vi "BCU诊断标定.vi"(8 "CAN端口":u16(ring), 9 "设备索引号":u16(ring), 10 "CAN卡类型":u32(ring)=21, 11 "Myindex":dbl=1.0) -> (3 "成功":bool)   [LabVIEW 2013] (continued)
                                frame "SOH" {
                                n3888 = control-ref of="SOH(%)"() -> (w5508:refnum<vi>)
                                n3889 = property class="DigNum (严格)"(reference=w5508, "Value"=0.0 ("值")) -> ()  [unwired: 1 in, 2 out]
                                }
                                frame "一级故障阀值" {
                                n3890 = local write "一级故障"(T10 {"总电压过高"=0.0, "整组电压不均衡"=0.0, "SOC过高"=0.0, "单体电压过高"=0.0, "总电压过低"=0.0, "温度过高"=0.0, "温度过低"=0.0, "单组电压不均衡"=0.0, "整组温度不均衡"=0.0, "单组温度不均衡"=0.0, "单体电压过低"=0.0, "充电电流过高"=0.0, "放电电流过高"=0.0, "SOC过低"=0.0, "内阻过大"=0.0, "极柱温度过高"=0.0, "SOH过低"=0.0} ("一级故障")) -> ()
                                }
                                frame "二级故障阀值" {
                                n3891 = local write "一级故障 2"(T10 {"总电压过高"=0.0, "整组电压不均衡"=0.0, "SOC过高"=0.0, "单体电压过高"=0.0, "总电压过低"=0.0, "温度过高"=0.0, "温度过低"=0.0, "单组电压不均衡"=0.0, "整组温度不均衡"=0.0, "单组温度不均衡"=0.0, "单体电压过低"=0.0, "充电电流过高"=0.0, "放电电流过高"=0.0, "SOC过低"=0.0, "内阻过大"=0.0, "极柱温度过高"=0.0, "SOH过低"=0.0} ("一级故障")) -> ()
                                }
                                frame "三级故障阀值" {
                                n3892 = local write "一级故障 3"(T10 {"总电压过高"=0.0, "整组电压不均衡"=0.0, "SOC过高"=0.0, "单体电压过高"=0.0, "总电压过低"=0.0, "温度过高"=0.0, "温度过低"=0.0, "单组电压不均衡"=0.0, "整组温度不均衡"=0.0, "单组温度不均衡"=0.0, "单体电压过低"=0.0, "充电电流过高"=0.0, "放电电流过高"=0.0, "SOC过低"=0.0, "内阻过大"=0.0, "极柱温度过高"=0.0, "SOH过低"=0.0} ("一级故障")) -> ()
                                }
                                frame "加热控制参数" {
                                n3893 = local write "加热控制参数"(T11 {"风机开启温度"=0.0, "风机关闭温度"=0.0, "加热开启温度"=0.0, "加热关闭温度"=0.0, "风机开启温差"=0.0, "风机关闭温差"=0.0, "加热关闭温差"=0.0} ("加热控制参数")) -> ()
                                }
                                frame "充电控制参数" {
                                n3894 = local write "一级故障 5"(T12 {"最大允许单体电压"=0.0, "最大允许总电压"=0.0, "最小允许单体电压"=0.0, "最大允许充电电流"=0.0, "最小允许充电电流"=0.0, "最大允许充电温度"=0.0, "最小允许充电温度"=0.0, "电流步长"=0.0} ("一级故障 5")) -> ()
                                }
                                frame "电池信息1" {
                                w5514 = ""
                                w5515 = 0.0 ("电池串联")
                                n3895 = local read "电池信息"() -> (w5517:T13)
                                n3896 = Bundle By Name(cluster=w5517, "电池串联"=w5515, "电池并联"=w5515, "电池包额定容量"=w5515, "电池包额定能量(kWh)"=w5515, "电池包额定总电压"=w5515, "实际容量"=w5515, "电池厂家"=w5514, "电池类型"=w5514, "电池生产日期"=w5514) -> (w5516:T13)
                                n3897 = local write "电池信息"(w5516) -> ()
                                }
                                frame "电池包组号" {
                                n3898 = local read "电池信息"() -> (w5520:T13)
                                n3899 = Bundle By Name(cluster=w5520, "电池包组号"="") -> (w5519:T13)
                                n3900 = local write "电池信息"(w5519) -> ()
                                }
                                frame "充放电安时" {
                                w5521 = 0.0 ("累计充电总安时")
                                n3901 = local read "电池信息"() -> (w5523:T13)
                                n3902 = Bundle By Name(cluster=w5523, "累计充电总安时"=w5521, "累计放电总安时"=w5521) -> (w5522:T13)
                                n3903 = local write "电池信息"(w5522) -> ()
                                }
                                frame "电池充放电次数" {
                                w5524 = 0.0 ("累计充电总安时")
                                n3904 = local read "电池信息"() -> (w5526:T13)
                                n3905 = Bundle By Name(cluster=w5526, "电池充满次数"=w5524, "电池放空次数"=w5524, "电池充电次数"=w5524) -> (w5525:T13)
                                n3906 = local write "电池信息"(w5525) -> ()
                                }
                                }
                              }
                              frame "从板" {
                                n3907 = case shown="\"温度起始值\"" w5527 {
                                frame "假", Default {
                                }
                                frame "电压起始值" {
                                n3908 = for {
                                N: 1 -> [_]
                                tunnel: [""] -> w5532 mode=indexing
                                }
                                n3909 = control-ref of="项目信息 2"() -> (w5528:refnum<vi>)
                                n3910 = call "表格数据输入-8.6.vi"("行数"=u32 0, "列数"=u32 1, "字符串数组"=w5532, "表格引用"=w5528) -> ()  [unwired: 8 in]
                                }
                                frame "通道电压个数" {
                                n3911 = for {
                                N: 5 -> [_]
                                tunnel: [""] -> w5538 mode=indexing
                                }
                                n3912 = control-ref of="项目信息 2"() -> (w5534:refnum<vi>)
                                n3913 = call "表格数据输入-8.6.vi"("行数"=u32 22, "列数"=u32 1, "字符串数组"=w5538, "表格引用"=w5534) -> ()  [unwired: 8 in]
                                }
                                frame "保险位置" {
                                n3914 = for {
                                N: 10 -> [_]
                                tunnel: [""] -> w5544 mode=indexing
                                }
                                n3915 = control-ref of="项目信息 2"() -> (w5540:refnum<vi>)
                                n3916 = call "表格数据输入-8.6.vi"("行数"=u32 2, "列数"=u32 1, "字符串数组"=w5544, "表格引用"=w5540) -> ()  [unwired: 8 in]
                                }
                                frame "温度起始值" {
                                n3917 = for {
                                N: 1 -> [_]
                                tunnel: [""] -> w5550 mode=indexing
                                }
                                n3918 = control-ref of="项目信息 2"() -> (w5546:refnum<vi>)
                                n3919 = call "表格数据输入-8.6.vi"("行数"=u32 1, "列数"=u32 1, "字符串数组"=w5550, "表格引用"=w5546) -> ()  [unwired: 8 in]
                                }
                                frame "加热控制参数" {
                                n3920 = local write "加热控制参数"(T11 {"风机开启温度"=0.0, "风机关闭温度"=0.0, "加热开启温度"=0.0, "加热关闭温度"=0.0, "风机开启温差"=0.0, "风机关闭温差"=0.0, "加热关闭温差"=0.0} ("加热控制参数")) -> ()
                                }
                                frame "一级故障阀值" {
                                n3921 = local write "一级故障 6"(T15 {"电压过高"=0.0, "电压过低"=0.0, "温度过高"=0.0, "温度过低"=0.0, "电压不均衡(V)"=0.0, "温度不均衡"=0.0, "SOC过低"=0.0} ("一级故障 6")) -> ()
                                }
                                frame "二级故障阀值" {
                                n3922 = local write "一级故障 7"(T15 {"电压过高"=0.0, "电压过低"=0.0, "温度过高"=0.0, "温度过低"=0.0, "电压不均衡(V)"=0.0, "温度不均衡"=0.0, "SOC过低"=0.0} ("一级故障 7")) -> ()
                                }
                                frame "三级故障阀值" {
                                n3923 = local write "一级故障 8"(T15 {"电压过高"=0.0, "电压过低"=0.0, "温度过高"=0.0, "温度过低"=0.0, "电压不均衡(V)"=0.0, "温度不均衡"=0.0, "SOC过低"=0.0} ("一级故障 7")) -> ()
                                }
                                frame "均衡参数" {
                                n3924 = local write "均衡参数"(T17 {"充电结束电压(90%)"=0.0, "充电结束电压(91%)"=0.0, "充电结束电压(92%)"=0.0, "充电结束电压(93%)"=0.0, "充电结束电压(94%)"=0.0, "均衡计算-电压高阀值1级"=0.0, "均衡计算-电压高阀值2级"=0.0, "均衡计算-电压低阀值1级"=0.0, "均衡计算-电压低阀值2级"=0.0, "均衡计算-最低电压阀值"=0.0, "均衡停止-最低电压阀值"=0.0, "均衡计算-电压极差阀值"=0.0, "充电结束电压(95%)"=0.0, "充电结束电压(96%)"=0.0, "充电结束电压(97%)"=0.0, "充电结束电压(98%)"=0.0, "充电结束电压(99%)"=0.0, "充电结束电压(100%)"=0.0} ("均衡参数")) -> ()
                                }
                                frame "均衡阀值" {
                                w5557 = sgl 0.0 ("均衡计算-电压高阀值1级")
                                n3925 = local read "均衡参数"() -> (w5558:T17)
                                n3926 = Bundle By Name(cluster=w5558, "均衡计算-电压高阀值1级"=w5557, "均衡计算-电压高阀值2级"=w5557, "均衡计算-电压低阀值1级"=w5557, "均衡计算-电压低阀值2级"=w5557, "均衡计算-最低电压阀值"=w5557, "均衡停止-最低电压阀值"=w5557, "均衡计算-电压极差阀值"=w5557) -> (w5559:T17)
                                n3927 = local write "均衡参数"(w5559) -> ()
                                }
                                frame "充电结束电压" {
                                w5560 = sgl 0.0 ("均衡计算-电压高阀值1级")
                                n3928 = local read "均衡参数"() -> (w5561:T17)
                                n3929 = Bundle By Name(cluster=w5561, "充电结束电压(90%)"=w5560, "充电结束电压(91%)"=w5560, "充电结束电压(92%)"=w5560, "充电结束电压(93%)"=w5560, "充电结束电压(94%)"=w5560, "充电结束电压(95%)"=w5560, "充电结束电压(96%)"=w5560, "充电结束电压(97%)"=w5560, "充电结束电压(98%)"=w5560, "充电结束电压(99%)"=w5560, "充电结束电压(100%)"=w5560) -> (w5562:T17)
                                n3930 = local write "均衡参数"(w5562) -> ()
                                }
                                }
                              }
                            }
                          }
                          frame #1 {
                            w5563 = FALSE ("流控帧")
                            w5564 = TRUE ("流控帧 2")
                            n3931 = global write "EV05全局变量1.vi" "写入超时"(w5563) -> ()
                            n3932 = global write "EV05全局变量1.vi" "流控帧"(w5563) -> ()
                            n3933 = local write "写?"(w5563) -> ()
                            n3934 = local write "消除"(w5564) -> ()
                            n3935 = local write "控制1"(w5564) -> ()
                            n3936 = global write "EV05全局变量1.vi" "流控帧 2"(w5564) -> ()
                          }
                          frame #2 {
                            n3937 = Wait Until Next ms Multiple(millisecond multiple=u32 300 ("毫秒倍数")) -> ()  [unwired: 1 out]
                          }
                          frame #3 {
                            n3938 = local read "设备索引号"() -> (w5567:u16)
                            n3939 = local read "CAN卡类型"() -> (w5568:u32)
                            n3940 = local read "CAN端口"() -> (w5566:u16)
                            n3941 = local write "命令序号"(w5571) -> ()
                            n3942 = stacked-sequence {
                              tunnel: w5572 -> [_ w5579]
                              tunnel: w5571 -> [_ w5578]
                              tunnel: w5570 -> [_ w5577]
                              tunnel: w5569 -> [_ w5576]
                              tunnel: w5568 -> [_ w5575]
                              tunnel: w5567 -> [_ w5574]
                              tunnel: w5566 -> [_ w5573]
                              frame #0 {
                              }
                              frame #1 {
                                n3943 = call "多帧发送机制(EV05).vi"("can卡类型"=w5575, "设备索引号"=w5574, "CAN端口"=w5573, "命令"=w5579, "板号"=w5577, "命令序号"=w5578, "输入数据"=w5576) -> ()  [unwired: 2 in, 11 out]
                              }
                            }
                          }
                          frame #4 {
                            n3944 = while {
                              tunnel: [w5584] -> w5581
                              tunnel: [w5583] -> w5580
                              i -> [w5587]
                              stop <- w5584 stop-if-true
                              n3945 = local read "强制终止读写标记"() -> (w5582:bool)
                              n3946 = global read "EV05全局变量1.vi" "写入超时"() -> (w5583:bool)
                              n3947 = Greater Or Equal?(x=w5587, y=20) -> (x >= y?=w5585:bool)
                              n3948 = Compound Arithmetic op=OR(w5582, w5583, w5585) -> (w5584:bool)
                              n3949 = Wait Until Next ms Multiple(millisecond multiple=u32 100 ("毫秒倍数")) -> ()  [unwired: 1 out]
                            }
                          }
                          frame #5 {
                            n3950 = case shown="假" w5596 {
                              tunnel: w5595 -> [w5607 _]
                              tunnel: [w5602 w5619] -> w5594
                              tunnel: w5593 -> [w5601 _]
                              tunnel: w5592 -> [w5600 w5619]
                              tunnel: [w5599 w5618] -> w5589
                              tunnel: w5591 -> [w5598 _]
                              tunnel: w5590 -> [w5597 w5618]
                              frame False {
                                n3951 = local read "重试次数"() -> (w5606:u8)
                                n3952 = Increment(x=w5606) -> (x+1=w5605:u8)
                                n3953 = local write "重试次数"(w5605) -> ()
                                n3954 = Greater Or Equal?(x=w5605, y=u8 4) -> (x >= y?=w5604:bool)
                                n3955 = case shown="真" w5604 {
                                tunnel: w5607 -> [_ w5612]
                                tunnel: [w5609 w5611] -> w5602
                                tunnel: w5601 -> [w5609 _]
                                tunnel: w5600 -> [_ w5611]
                                tunnel: [w5608 w5610] -> w5599
                                tunnel: w5598 -> [w5608 _]
                                tunnel: w5597 -> [_ w5610]
                                frame False {
                                }
                                frame True {
                                n3956 = control-ref of="结果"() -> (w5614:refnum<vi>)
                                n3957 = Concatenate Strings(w5612, "     读取失败" ("字符串")) -> (w5616:string)
                                n3958 = Build Array(w5616) -> (w5613:string[])
                                n3959 = call "表格编辑.vi"("新元素/子数组"=w5613, "活动单元格:单元格背景色"=u32 16740749, "MCListbox引用句柄"=w5614) -> ()  [unwired: 9 out]
                                }
                                }
                              }
                              frame True {
                              }
                            }
                          }
                          frame #6 {
                            n3960 = And(x=w5621, y=w5623) -> (x .and. y?=w5622:bool)
                            n3961 = case shown="真" w5622 {
                              frame False {
                              }
                              frame True {
                                n3962 = local write "强制终止读写标记"(FALSE ("强制停止")) -> ()
                                n3963 = control-ref of="结果"() -> (w5626:refnum<vi>)
                                n3964 = Concatenate Strings("读取完成" ("字符串")) -> (w5628:string)
                                n3965 = Build Array(w5628) -> (w5625:string[])
                                n3966 = call "表格编辑.vi"("新元素/子数组"=w5625, "活动单元格:单元格背景色"=u32 21937, "MCListbox引用句柄"=w5626) -> ()  [unwired: 9 out]
                              }
                            }
                            n3967 = Wait (ms)(milliseconds to wait=u32 50 ("等待时间（毫秒）")) -> ()  [unwired: 1 out]
                          }
                        }
                      }
                    }
                  }
                  n3968 = local read "强制终止读写标记"() -> (w5394:bool)
                  n3969 = Or(x=w5394, y=w5393) -> (x .or. y?=w5391:bool)
                }
              }
            }
            frame #2 {
              n3970 = case shown="假" w5713 {
                tunnel: w5714 -> [w5715 _]
                frame False {
                  n3971 = case shown="\"主板\", 默认" w5715 {
                    frame "主板", Default {
                      n3972 = global read "读配置文件全局.vi" "电池额定实际容量判定"() -> (w5729:bool)
                      n3973 = global read "读配置文件全局.vi" "电池充放电次数判定"() -> (w5718:bool)
                      n3974 = global read "读配置文件全局.vi" "加热控制参数判定"() -> (w5716:bool)
                      n3975 = global read "读配置文件全局.vi" "配置文件版本判定"() -> (w5728:bool)
                      n3976 = global read "读配置文件全局.vi" "充电控制参数判定"() -> (w5722:bool)
                      n3977 = global read "读配置文件全局.vi" "通道电压数判定"() -> (w5734:bool)
                      n3978 = global read "读配置文件全局.vi" "电压起始值判定"() -> (w5733:bool)
                      n3979 = global read "读配置文件全局.vi" "温度起始值判定"() -> (w5731:bool)
                      n3980 = global read "读配置文件全局.vi" "充放电安时判定"() -> (w5720:bool)
                      n3981 = global read "读配置文件全局.vi" "电池包组号判定"() -> (w5719:bool)
                      n3982 = global read "读配置文件全局.vi" "电池信息1判定"() -> (w5721:bool)
                      n3983 = global read "读配置文件全局.vi" "从板个数判定"() -> (w5737:bool)
                      n3984 = global read "读配置文件全局.vi" "产品编号判定"() -> (w5736:bool)
                      n3985 = global read "读配置文件全局.vi" "电压个数判定"() -> (w5735:bool)
                      n3986 = global read "读配置文件全局.vi" "温度个数判定"() -> (w5732:bool)
                      n3987 = global read "读配置文件全局.vi" "保险位置判定"() -> (w5730:bool)
                      n3988 = global read "读配置文件全局.vi" "一级故障判定"() -> (w5725:bool)
                      n3989 = global read "读配置文件全局.vi" "二级故障判定"() -> (w5724:bool)
                      n3990 = global read "读配置文件全局.vi" "三级故障判定"() -> (w5723:bool)
                      n3991 = global read "读配置文件全局.vi" "车牌号判定"() -> (w5727:bool)
                      n3992 = global read "读配置文件全局.vi" "SOH判定"() -> (w5726:bool)
                      n3993 = Build Array(w5737, w5736, w5735, w5734, w5733, w5732, w5731, w5730, w5729, w5728, w5727, w5726, w5725, w5724, w5723, w5722, w5721, w5720, w5719, w5718, w5716) -> (w5717:bool[])
                      n3994 = And Array Elements(Boolean array=w5717) -> (logical AND=w5738:bool)
                      n3995 = disable-structure shown="禁用" {
                        frame Disabled {
                          n3996 = global read "读配置文件全局.vi" "SOC判定"() -> ()  [unwired: 1 out]
                        }
                        frame Enabled {
                        }
                      }
                      n3997 = case shown="假" w5738 {
                        tunnel: w5717 -> [_ w5743]
                        frame True {
                          n3998 = control-ref of="结果"() -> (w5741:refnum<vi>)
                          n3999 = Build Array("全部判定成功!!!!!!!!") -> (w5742:string[])
                          n4000 = call "表格编辑.vi"("新元素/子数组"=w5742, "活动单元格:单元格背景色"=u32 6618880, "MCListbox引用句柄"=w5741) -> ()  [unwired: 9 out]
                        }
                        frame False {
                          n4001 = stacked-sequence {
                            tunnel: w5743 -> [_ w5748]
                            frame #0 {
                              n4002 = control-ref of="结果"() -> (w5746:refnum<vi>)
                              n4003 = Build Array("全部判定失败!!!!!") -> (w5747:string[])
                              n4004 = call "表格编辑.vi"("新元素/子数组"=w5747, "活动单元格:单元格背景色"=u32 16711680, "MCListbox引用句柄"=w5746) -> ()  [unwired: 9 out]
                            }
                            frame #1 {
                              n4005 = for {
                                tunnel: w5748 -> [w5750] mode=indexing
                                i -> [w5749]
                                n4006 = case shown="20" w5749 {
                                tunnel: w5750 -> [w5751 w5756 w5761 w5766 w5771 w5776 w5781 w5786 w5791 w5796 w5801 w5806 w5811 w5816 w5821 w5826 w5831 w5836 w5841 w5846 w5851 _]
                                frame 0 {
                                n4007 = case shown="假" w5751 {
                                frame False {
                                n4008 = control-ref of="结果"() -> (w5754:refnum<vi>)
                                n4009 = Build Array("从板个数判定失败!") -> (w5755:string[])
                                n4010 = call "表格编辑.vi"("新元素/子数组"=w5755, "活动单元格:单元格背景色"=u32 16711680, "MCListbox引用句柄"=w5754) -> ()  [unwired: 9 out]
                                }
                                frame True {
                                }
                                }
                                }
                                frame 1 {
                                n4011 = case shown="假" w5756 {
                                frame False {
                                n4012 = control-ref of="结果"() -> (w5759:refnum<vi>)
                                n4013 = Build Array("产品编号判定失败!") -> (w5760:string[])
                                n4014 = call "表格编辑.vi"("新元素/子数组"=w5760, "活动单元格:单元格背景色"=u32 16711680, "MCListbox引用句柄"=w5759) -> ()  [unwired: 9 out]
                                }
                                frame True {
                                }
                                }
                                }
                                frame 2 {
                                n4015 = case shown="假" w5761 {
                                frame False {
                                n4016 = control-ref of="结果"() -> (w5764:refnum<vi>)
                                n4017 = Build Array("电压个数判定失败!") -> (w5765:string[])
                                n4018 = call "表格编辑.vi"("新元素/子数组"=w5765, "活动单元格:单元格背景色"=u32 16711680, "MCListbox引用句柄"=w5764) -> ()  [unwired: 9 out]
                                }
                                frame True {
                                }
                                }
                                }
                                frame 3 {
                                n4019 = case shown="假" w5766 {
                                frame False {
                                n4020 = control-ref of="结果"() -> (w5769:refnum<vi>)
                                n4021 = Build Array("通道电压数判定失败!") -> (w5770:string[])
                                n4022 = call "表格编辑.vi"("新元素/子数组"=w5770, "活动单元格:单元格背景色"=u32 16711680, "MCListbox引用句柄"=w5769) -> ()  [unwired: 9 out]
                                }
                                frame True {
                                }
                                }
                                }
                                frame 4 {
                                n4023 = case shown="假" w5771 {
                                frame False {
                                n4024 = control-ref of="结果"() -> (w5774:refnum<vi>)
                                n4025 = Build Array("电压起始值判定失败!") -> (w5775:string[])
                                n4026 = call "表格编辑.vi"("新元素/子数组"=w5775, "活动单元格:单元格背景色"=u32 16711680, "MCListbox引用句柄"=w5774) -> ()  [unwired: 9 out]
                                }
                                frame True {
                                }
                                }
                                }
                                frame 5 {
                                n4027 = case shown="假" w5776 {
                                frame False {
                                n4028 = control-ref of="结果"() -> (w5779:refnum<vi>)
                                n4029 = Build Array("温度个数判定失败!") -> (w5780:string[])
                                n4030 = call "表格编辑.vi"("新元素/子数组"=w5780, "活动单元格:单元格背景色"=u32 16711680, "MCListbox引用句柄"=w5779) -> ()  [unwired: 9 out]
                                }
                                frame True {
                                }
                                }
                                }
                                frame 6 {
                                n4031 = case shown="假" w5781 {
                                frame False {
                                n4032 = control-ref of="结果"() -> (w5784:refnum<vi>)
                                n4033 = Build Array("温度起始值判定失败!") -> (w5785:string[])
                                n4034 = call "表格编辑.vi"("新元素/子数组"=w5785, "活动单元格:单元格背景色"=u32 16711680, "MCListbox引用句柄"=w5784) -> ()  [unwired: 9 out]
                                }
                                frame True {
                                }
                                }
                                }
                                frame 7 {
                                n4035 = case shown="假" w5786 {
                                frame False {
                                n4036 = control-ref of="结果"() -> (w5789:refnum<vi>)
                                n4037 = Build Array("保险位置判定失败!") -> (w5790:string[])
                                n4038 = call "表格编辑.vi"("新元素/子数组"=w5790, "活动单元格:单元格背景色"=u32 16711680, "MCListbox引用句柄"=w5789) -> ()  [unwired: 9 out]
                                }
                                frame True {
                                }
                                }
                                }
                                frame 8 {
                                n4039 = case shown="假" w5791 {
                                frame False {
                                n4040 = control-ref of="结果"() -> (w5794:refnum<vi>)
                                n4041 = Build Array("电池额定实际容量判定失败!") -> (w5795:string[])
                                n4042 = call "表格编辑.vi"("新元素/子数组"=w5795, "活动单元格:单元格背景色"=u32 16711680, "MCListbox引用句柄"=w5794) -> ()  [unwired: 9 out]
                                }
                                frame True {
                                }
                                }
                                }
                                frame 9 {
                                n4043 = case shown="假" w5796 {
                                frame False {
                                n4044 = control-ref of="结果"() -> (w5799:refnum<vi>)
                                n4045 = Build Array("配置文件版本判定失败!") -> (w5800:string[])
                                n4046 = call "表格编辑.vi"("新元素/子数组"=w5800, "活动单元格:单元格背景色"=u32 16711680, "MCListbox引用句柄"=w5799) -> ()  [unwired: 9 out]
                                }
                                frame True {
                                }
                                }
                                }
                                frame 10 {
                                n4047 = case shown="假" w5801 {
                                frame False {
                                n4048 = control-ref of="结果"() -> (w5804:refnum<vi>)
                                n4049 = Build Array("车牌号判定失败!") -> (w5805:string[])
                                n4050 = call "表格编辑.vi"("新元素/子数组"=w5805, "活动单元格:单元格背景色"=u32 16711680, "MCListbox引用句柄"=w5804) -> ()  [unwired: 9 out]
                                }
                                frame True {
                                }
                                }
                                }
                                frame 11 {
                                n4051 = case shown="假" w5806 {
                                frame False {
                                n4052 = control-ref of="结果"() -> (w5809:refnum<vi>)
                                n4053 = Build Array("SOH判定失败!") -> (w5810:string[])
                                n4054 = call "表格编辑.vi"("新元素/子数组"=w5810, "活动单元格:单元格背景色"=u32 16711680, "MCListbox引用句柄"=w5809) -> ()  [unwired: 9 out]
                                }
                                frame True {
                                }
                                }
                                }
                                frame 12 {
                                n4055 = case shown="假" w5811 {
                                frame False {
                                n4056 = control-ref of="结果"() -> (w5814:refnum<vi>)
                                n4057 = Build Array("一级故障阀值判定失败!") -> (w5815:string[])
                                n4058 = call "表格编辑.vi"("新元素/子数组"=w5815, "活动单元格:单元格背景色"=u32 16711680, "MCListbox引用句柄"=w5814) -> ()  [unwired: 9 out]
                                }
                                frame True {
                                }
                                }
                                }
                                frame 13 {
                                n4059 = case shown="假" w5816 {
                                frame False {
                                n4060 = control-ref of="结果"() -> (w5819:refnum<vi>)
                                n4061 = Build Array("二级故障阀值判定失败!") -> (w5820:string[])
                                n4062 = call "表格编辑.vi"("新元素/子数组"=w5820, "活动单元格:单元格背景色"=u32 16711680, "MCListbox引用句柄"=w5819) -> ()  [unwired: 9 out]
                                }
                                frame True {
                                }
                                }
                                }
                                frame 14 {
                                n4063 = case shown="假" w5821 {
                                frame False {
                                n4064 = control-ref of="结果"() -> (w5824:refnum<vi>)
                                n4065 = Build Array("三级故障阀值判定失败!") -> (w5825:string[])
                                n4066 = call "表格编辑.vi"("新元素/子数组"=w5825, "活动单元格:单元格背景色"=u32 16711680, "MCListbox引用句柄"=w5824) -> ()  [unwired: 9 out]
                                }
                                frame True {
                                }
                                }
                                }
                                frame 15 {
                                n4067 = case shown="假" w5826 {
                                frame False {
                                n4068 = control-ref of="结果"() -> (w5829:refnum<vi>)
                                n4069 = Build Array("充电控制参数判定失败!") -> (w5830:string[])
                                n4070 = call "表格编辑.vi"("新元素/子数组"=w5830, "活动单元格:单元格背景色"=u32 16711680, "MCListbox引用句柄"=w5829) -> ()  [unwired: 9 out]
                                }
                                frame True {
                                }
                                }
                                }
                                frame 16 {
                                n4071 = case shown="假" w5831 {
                                frame False {
                                n4072 = control-ref of="结果"() -> (w5834:refnum<vi>)
                                n4073 = Build Array("电池信息1判定失败!") -> (w5835:string[])
                                n4074 = call "表格编辑.vi"("新元素/子数组"=w5835, "活动单元格:单元格背景色"=u32 16711680, "MCListbox引用句柄"=w5834) -> ()  [unwired: 9 out]
                                }
                                frame True {
                                }
                                }
                                }
                                frame 17 {
                                n4075 = case shown="假" w5836 {
                                frame False {
                                n4076 = control-ref of="结果"() -> (w5839:refnum<vi>)
                                n4077 = Build Array("充放电安时判定失败!") -> (w5840:string[])
                                n4078 = call "表格编辑.vi"("新元素/子数组"=w5840, "活动单元格:单元格背景色"=u32 16711680, "MCListbox引用句柄"=w5839) -> ()  [unwired: 9 out]
                                }
                                frame True {
                                }
                                }
                                }
                                frame 18 {
                                n4079 = case shown="假" w5841 {
                                frame False {
                                n4080 = control-ref of="结果"() -> (w5844:refnum<vi>)
                                n4081 = Build Array("电池包组号判定失败!") -> (w5845:string[])
                                n4082 = call "表格编辑.vi"("新元素/子数组"=w5845, "活动单元格:单元格背景色"=u32 16711680, "MCListbox引用句柄"=w5844) -> ()  [unwired: 9 out]
                                }
                                frame True {
                                }
                                }
                                }
                                frame 19 {
                                n4083 = case shown="假" w5846 {
                                frame False {
                                n4084 = control-ref of="结果"() -> (w5849:refnum<vi>)
                                n4085 = Build Array("电池充放电次数判定失败!") -> (w5850:string[])
                                n4086 = call "表格编辑.vi"("新元素/子数组"=w5850, "活动单元格:单元格背景色"=u32 16711680, "MCListbox引用句柄"=w5849) -> ()  [unwired: 9 out]
                                }
                                frame True {
                                }
                                }
                                }
                                frame 20 {
                                n4087 = case shown="假" w5851 {
                                frame False {
                                n4088 = control-ref of="结果"() -> (w5854:refnum<vi>)
                                n4089 = Build Array("加热控制参数判定失败!") -> (w5855:string[])
                                n4090 = call "表格编辑.vi"("新元素/子数组"=w5855, "活动单元格:单元格背景色"=u32 16711680, "MCListbox引用句柄"=w5854) -> ()  [unwired: 9 out]
                                }
                                frame True {
                                }
                                }
                                }
                                frame 99, Default {
                                }
                                }
                              }
                            }
                          }
                        }
                      }
                    }
                    frame "从板" {
                      n4091 = global read "读配置文件全局2.vi" "电压起始值判定"() -> (w5864:bool)
                      n4092 = global read "读配置文件全局2.vi" "温度起始值判定"() -> (w5861:bool)
                      n4093 = global read "读配置文件全局2.vi" "加热控制参数判定"() -> (w5856:bool)
                      n4094 = global read "读配置文件全局2.vi" "通道电压判定"() -> (w5863:bool)
                      n4095 = global read "读配置文件全局2.vi" "保险位置判定"() -> (w5862:bool)
                      n4096 = global read "读配置文件全局2.vi" "一级故障判定"() -> (w5859:bool)
                      n4097 = global read "读配置文件全局2.vi" "二级故障判定"() -> (w5858:bool)
                      n4098 = global read "读配置文件全局2.vi" "三级故障判定"() -> (w5857:bool)
                      n4099 = global read "读配置文件全局2.vi" "从板号判定"() -> (w5865:bool)
                      n4100 = Build Array(w5865, w5864, w5863, w5862, w5861, w5859, w5858, w5857, w5856) -> (w5860:bool[])
                      n4101 = And Array Elements(Boolean array=w5860) -> (logical AND=w5866:bool)
                      n4102 = case shown="假" w5866 {
                        tunnel: w5860 -> [_ w5871]
                        frame True {
                          n4103 = control-ref of="结果"() -> (w5869:refnum<vi>)
                          n4104 = Build Array("读取判定成功!!!!!!!!") -> (w5870:string[])
                          n4105 = call "表格编辑.vi"("新元素/子数组"=w5870, "活动单元格:单元格背景色"=u32 6618880, "MCListbox引用句柄"=w5869) -> ()  [unwired: 9 out]
                        }
                        frame False {
                          n4106 = stacked-sequence {
                            tunnel: w5871 -> [_ w5876]
                            frame #0 {
                              n4107 = control-ref of="结果"() -> (w5874:refnum<vi>)
                              n4108 = Build Array("读取判定失败!!!!!") -> (w5875:string[])
                              n4109 = call "表格编辑.vi"("新元素/子数组"=w5875, "活动单元格:单元格背景色"=u32 16711680, "MCListbox引用句柄"=w5874) -> ()  [unwired: 9 out]
                            }
                            frame #1 {
                              n4110 = for {
                                tunnel: w5876 -> [w5877] mode=indexing
                                i -> [w5878]
                                n4111 = case shown="0" w5878 {
                                tunnel: w5877 -> [w5879 w5884 w5889 w5894 w5899 w5904 w5909 w5914 w5919 _]
                                frame 0 {
                                n4112 = case shown="假" w5879 {
                                frame False {
                                n4113 = control-ref of="结果"() -> (w5882:refnum<vi>)
                                n4114 = Build Array("从板号判定失败!") -> (w5883:string[])
                                n4115 = call "表格编辑.vi"("新元素/子数组"=w5883, "活动单元格:单元格背景色"=u32 16711680, "MCListbox引用句柄"=w5882) -> ()  [unwired: 9 out]
                                }
                                frame True {
                                }
                                }
                                }
                                frame 1 {
                                n4116 = case shown="假" w5884 {
                                frame False {
                                n4117 = control-ref of="结果"() -> (w5887:refnum<vi>)
                                n4118 = Build Array("电压起始值判定失败!") -> (w5888:string[])
                                n4119 = call "表格编辑.vi"("新元素/子数组"=w5888, "活动单元格:单元格背景色"=u32 16711680, "MCListbox引用句柄"=w5887) -> ()  [unwired: 9 out]
                                }
                                frame True {
                                }
                                }
                                }
                                frame 2 {
                                n4120 = case shown="假" w5889 {
                                frame False {
                                n4121 = control-ref of="结果"() -> (w5892:refnum<vi>)
                                n4122 = Build Array("通道电压节数判定失败!") -> (w5893:string[])
                                n4123 = call "表格编辑.vi"("新元素/子数组"=w5893, "活动单元格:单元格背景色"=u32 16711680, "MCListbox引用句柄"=w5892) -> ()  [unwired: 9 out]
                                }
                                frame True {
                                }
                                }
                                }
                                frame 3 {
                                n4124 = case shown="假" w5894 {
                                frame False {
                                n4125 = control-ref of="结果"() -> (w5897:refnum<vi>)
                                n4126 = Build Array("保险位置判定失败!") -> (w5898:string[])
                                n4127 = call "表格编辑.vi"("新元素/子数组"=w5898, "活动单元格:单元格背景色"=u32 16711680, "MCListbox引用句柄"=w5897) -> ()  [unwired: 9 out]
                                }
                                frame True {
                                }
                                }
                                }
                                frame 4 {
                                n4128 = case shown="假" w5899 {
                                frame False {
                                n4129 = control-ref of="结果"() -> (w5902:refnum<vi>)
                                n4130 = Build Array("温度起始值判定失败!") -> (w5903:string[])
                                n4131 = call "表格编辑.vi"("新元素/子数组"=w5903, "活动单元格:单元格背景色"=u32 16711680, "MCListbox引用句柄"=w5902) -> ()  [unwired: 9 out]
                                }
                                frame True {
                                }
                                }
                                }
                                frame 5 {
                                n4132 = case shown="假" w5904 {
                                frame False {
                                n4133 = control-ref of="结果"() -> (w5907:refnum<vi>)
                                n4134 = Build Array("一级故障判定失败!") -> (w5908:string[])
                                n4135 = call "表格编辑.vi"("新元素/子数组"=w5908, "活动单元格:单元格背景色"=u32 16711680, "MCListbox引用句柄"=w5907) -> ()  [unwired: 9 out]
                                }
                                frame True {
                                }
                                }
                                }
                                frame 6 {
                                n4136 = case shown="假" w5909 {
                                frame False {
                                n4137 = control-ref of="结果"() -> (w5912:refnum<vi>)
                                n4138 = Build Array("二级故障判定失败!") -> (w5913:string[])
                                n4139 = call "表格编辑.vi"("新元素/子数组"=w5913, "活动单元格:单元格背景色"=u32 16711680, "MCListbox引用句柄"=w5912) -> ()  [unwired: 9 out]
                                }
                                frame True {
                                }
                                }
                                }
                                frame 7 {
                                n4140 = case shown="假" w5914 {
                                frame False {
                                n4141 = control-ref of="结果"() -> (w5917:refnum<vi>)
                                n4142 = Build Array("三级故障判定失败!") -> (w5918:string[])
                                n4143 = call "表格编辑.vi"("新元素/子数组"=w5918, "活动单元格:单元格背景色"=u32 16711680, "MCListbox引用句柄"=w5917) -> ()  [unwired: 9 out]
                                }
                                frame True {
                                }
                                }
                                }
                                frame 8 {
                                n4144 = case shown="假" w5919 {
                                frame False {
                                n4145 = control-ref of="结果"() -> (w5922:refnum<vi>)
                                n4146 = Build Array("加热控制参数判定失败!") -> (w5923:string[])
                                n4147 = call "表格编辑.vi"("新元素/子数组"=w5923, "活动单元格:单元格背景色"=u32 16711680, "MCListbox引用句柄"=w5922) -> ()  [unwired: 9 out]
                                }
                                frame True {
                                }
                                }
                                }
                                frame 99, Default {
                                }
                                }
                              }
                            }
                          }
                        }
                      }
                      n4148 = disable-structure shown="禁用" {
                        frame Disabled {
                          n4149 = global read "读配置文件全局.vi" "SOC判定"() -> ()  [unwired: 1 out]
                        }
                        frame Enabled {
                        }
                      }
                    }
                  }
                }
                frame True {
                }
              }
            }
          }
          n4150 = stacked-sequence {
            tunnel: w5156 -> [_]
            frame #0 {
              n4151 = local write "强制终止读写标记"(FALSE ("强制停止")) -> ()
            }
          }
          "重试次数" <- u8 0 ("重试次数")
        }
        frame "开启均衡" {
          n4152 = local read "从板板号"() -> (w5924:u8)
          n4153 = stacked-sequence {
            tunnel: 133 -> [_ w5950 _ _]
            tunnel: w5924 -> [_ _ _ _]
            frame #0 {
              w5934 = u8 0 items=["Normal", "Listen Only"] ("工作方式")
              w5933 = u8 1 items=["Dual Filter", "Single Filter"] ("滤波方式")
              n4154 = global write "EV05全局变量1.vi" "读取超时"(FALSE ("读取超时")) -> ()
              n4155 = global write "EV05全局变量1.vi" "流控帧 2"(TRUE ("流控帧 2")) -> ()
              n4156 = local write "写?"(TRUE ("写?")) -> ()
              n4157 = local read "设备索引号"() -> (w5929:u16)
              n4158 = local read "CAN卡类型"() -> (w5928:u32)
              n4159 = local read "CAN端口"() -> (w5930:u16)
              n4160 = local write "控制1"(TRUE ("控制1")) -> ()
              n4161 = local write "消除"(TRUE ("消除")) -> ()
              n4162 = global write "EV05全局变量1.vi" "流控帧"(FALSE ("流控帧")) -> ()
              n4163 = call "CAN_Init-8.6.vi"("CAN卡类型"=w5928, "设备索引号"=w5929, "CAN端口"=w5930, "操作类型"=enum16{"初始化CAN", "关闭CAN"}."初始化CAN", "滤波方式"=w5933, "Accept Code"=u32 606601216, "簇"=T23 {"打开CAN"=FALSE, "初始化CAN"=TRUE, "开始CAN"=TRUE, "重启"=FALSE, "关闭CAN"=FALSE}, "Mask Code"=u32 524287 ("Accept Code"), "工作方式"=w5934, "是否滤波"=TRUE, "滤波选择"=T22 {"fiter_mode"=1, "fiter_endid"=75825152, "fiter_startid"=75890687}) -> ()  [unwired: 3 in, 6 out]
              n4164 = Wait Until Next ms Multiple(millisecond multiple=u32 20 ("毫秒倍数")) -> ()  [unwired: 1 out]
            }
            frame #1 {
              n4165 = local write "命令"(w5950) -> ()
              n4166 = call "ID组合.vi"("SA(4)"=0 ("PDU(1)"), "PS(3)"=63 ("PDU(1)"), "PF(2)"=w5950, "PDU(1)"=4) -> ("ID"=w5949:i32)  [unwired: 7 out]
              n4167 = local read "均衡类型选择"() -> (w5946:enum16{"放电均衡", "充电均衡", "充放电均衡"})
              n4168 = local read "设备索引号"() -> (w5955:u16)
              n4169 = local read "CAN卡类型"() -> (w5956:u32)
              n4170 = local read "CAN端口"() -> (w5954:u16)
              n4171 = local write "命令序号"(2) -> ()
              n4172 = Add(x=w5946, y=1) -> (x+y=w5944:i32)
              n4173 = Build Array(2, 2, w5944) -> (w5957:i32[])
              n4174 = call "transmit-8.6.vi"("can卡类型"=w5956, "设备索引号"=w5955, "CAN端口"=w5954, "ID"=w5949, "SendType"=u8 0, "Data"=w5957) -> ()  [unwired: 3 in, 11 out]
            }
            frame #2 {
              n4175 = Wait Until Next ms Multiple(millisecond multiple=u32 1000 ("毫秒倍数")) -> ()  [unwired: 1 out]
            }
            frame #3 {
              w5965 = u8 0 items=["Normal", "Listen Only"] ("工作方式")
              w5966 = u8 1 items=["Dual Filter", "Single Filter"] ("滤波方式")
              n4176 = global write "EV05全局变量1.vi" "流控帧 2"(FALSE ("流控帧 2")) -> ()
              n4177 = local read "CAN卡类型"() -> (w5971:u32)
              n4178 = local read "设备索引号"() -> (w5970:u16)
              n4179 = local read "CAN端口"() -> (w5969:u16)
              n4180 = local write "控制1"(FALSE ("控制1")) -> ()
              n4181 = local write "消除"(FALSE ("消除")) -> ()
              n4182 = call <vilib>:"Unset Busy.vi"() -> ()  [unwired: 2 in, 10 out]
              n4183 = call "CAN_Init-8.6.vi"("CAN卡类型"=w5971, "设备索引号"=w5970, "CAN端口"=w5969, "操作类型"=enum16{"初始化CAN", "关闭CAN"}."初始化CAN", "滤波方式"=w5966, "Accept Code"=u32 3221225472, "簇"=T23 {"打开CAN"=FALSE, "初始化CAN"=TRUE, "开始CAN"=TRUE, "重启"=FALSE, "关闭CAN"=FALSE}, "Mask Code"=u32 1073741823 ("Accept Code"), "工作方式"=w5965, "是否滤波"=TRUE, "滤波选择"=T22 {"fiter_mode"=1, "fiter_endid"=402653184, "fiter_startid"=419430399}) -> ()  [unwired: 3 in, 6 out]
            }
          }
        }
        frame "关闭均衡" {
          n4184 = local read "从板板号"() -> (w5975:u8)
          n4185 = stacked-sequence {
            tunnel: 133 -> [_ w5999 _ _]
            tunnel: w5975 -> [_ _ _ _]
            frame #0 {
              w5985 = u8 0 items=["Normal", "Listen Only"] ("工作方式")
              w5984 = u8 1 items=["Dual Filter", "Single Filter"] ("滤波方式")
              n4186 = global write "EV05全局变量1.vi" "读取超时"(FALSE ("读取超时")) -> ()
              n4187 = global write "EV05全局变量1.vi" "流控帧 2"(TRUE ("流控帧 2")) -> ()
              n4188 = local write "写?"(TRUE ("写?")) -> ()
              n4189 = local read "设备索引号"() -> (w5980:u16)
              n4190 = local read "CAN卡类型"() -> (w5979:u32)
              n4191 = local read "CAN端口"() -> (w5981:u16)
              n4192 = local write "控制1"(TRUE ("控制1")) -> ()
              n4193 = global write "EV05全局变量1.vi" "流控帧"(FALSE ("流控帧")) -> ()
              n4194 = local write "消除"(TRUE ("消除")) -> ()
              n4195 = call "CAN_Init-8.6.vi"("CAN卡类型"=w5979, "设备索引号"=w5980, "CAN端口"=w5981, "操作类型"=enum16{"初始化CAN", "关闭CAN"}."初始化CAN", "滤波方式"=w5984, "Accept Code"=u32 606601216, "簇"=T23 {"打开CAN"=FALSE, "初始化CAN"=TRUE, "开始CAN"=TRUE, "重启"=FALSE, "关闭CAN"=FALSE}, "Mask Code"=u32 524287 ("Accept Code"), "工作方式"=w5985, "是否滤波"=TRUE, "滤波选择"=T22 {"fiter_mode"=1, "fiter_endid"=75825152, "fiter_startid"=75890687}) -> ()  [unwired: 3 in, 6 out]
              n4196 = Wait Until Next ms Multiple(millisecond multiple=u32 20 ("毫秒倍数")) -> ()  [unwired: 1 out]
            }
            frame #1 {
              n4197 = local write "命令"(w5999) -> ()
              n4198 = call "ID组合.vi"("SA(4)"=0 ("PDU(1)"), "PS(3)"=63 ("PDU(1)"), "PF(2)"=w5999, "PDU(1)"=4) -> ("ID"=w5998:i32)  [unwired: 7 out]
              n4199 = local read "均衡类型选择"() -> (w6009:enum16{"放电均衡", "充电均衡", "充放电均衡"})
              n4200 = local write "命令序号"(3) -> ()
              n4201 = local read "设备索引号"() -> (w6004:u16)
              n4202 = local read "CAN卡类型"() -> (w6005:u32)
              n4203 = local read "CAN端口"() -> (w6003:u16)
              n4204 = Add(x=w6009, y=1) -> (x+y=w6007:i32)
              n4205 = Build Array(2, 3, w6007) -> (w6006:i32[])
              n4206 = call "transmit-8.6.vi"("can卡类型"=w6005, "设备索引号"=w6004, "CAN端口"=w6003, "ID"=w5998, "SendType"=u8 0, "Data"=w6006) -> ()  [unwired: 3 in, 11 out]
            }
            frame #2 {
              n4207 = Wait Until Next ms Multiple(millisecond multiple=u32 1000 ("毫秒倍数")) -> ()  [unwired: 1 out]
            }
            frame #3 {
              w6016 = u8 0 items=["Normal", "Listen Only"] ("工作方式")
              w6017 = u8 1 items=["Dual Filter", "Single Filter"] ("滤波方式")
              n4208 = local read "设备索引号"() -> (w6021:u16)
              n4209 = local read "CAN卡类型"() -> (w6022:u32)
              n4210 = global write "EV05全局变量1.vi" "流控帧 2"(FALSE ("流控帧 2")) -> ()
              n4211 = local read "CAN端口"() -> (w6020:u16)
              n4212 = local write "控制1"(FALSE ("控制1")) -> ()
              n4213 = local write "消除"(FALSE ("消除")) -> ()
              n4214 = call "CAN_Init-8.6.vi"("CAN卡类型"=w6022, "设备索引号"=w6021, "CAN端口"=w6020, "操作类型"=enum16{"初始化CAN", "关闭CAN"}."初始化CAN", "滤波方式"=w6017, "Accept Code"=u32 3221225472, "簇"=T23 {"打开CAN"=FALSE, "初始化CAN"=TRUE, "开始CAN"=TRUE, "重启"=FALSE, "关闭CAN"=FALSE}, "Mask Code"=u32 1073741823 ("Accept Code"), "工作方式"=w6016, "是否滤波"=TRUE, "滤波选择"=T22 {"fiter_mode"=1, "fiter_endid"=402653184, "fiter_startid"=419430399}) -> ()  [unwired: 3 in, 6 out]
              n4215 = call <vilib>:"Unset Busy.vi"() -> ()  [unwired: 2 in, 10 out]
            }
          }
        }
        frame "强制均衡" {
          n4216 = local read "从板板号"() -> (w6026:u8)
          n4217 = stacked-sequence {
            tunnel: 133 -> [_ w6057 _ _]
            tunnel: w6026 -> [_ _ _ _]
            frame #0 {
              w6036 = u8 0 items=["Normal", "Listen Only"] ("工作方式")
              w6035 = u8 1 items=["Dual Filter", "Single Filter"] ("滤波方式")
              n4218 = global write "EV05全局变量1.vi" "读取超时"(FALSE ("读取超时")) -> ()
              n4219 = global write "EV05全局变量1.vi" "流控帧 2"(TRUE ("流控帧 2")) -> ()
              n4220 = local write "写?"(TRUE ("写?")) -> ()
              n4221 = local read "设备索引号"() -> (w6031:u16)
              n4222 = local read "CAN卡类型"() -> (w6030:u32)
              n4223 = local write "控制1"(TRUE ("控制1")) -> ()
              n4224 = local read "CAN端口"() -> (w6032:u16)
              n4225 = local write "消除"(TRUE ("消除")) -> ()
              n4226 = global write "EV05全局变量1.vi" "流控帧"(FALSE ("流控帧")) -> ()
              n4227 = call "CAN_Init-8.6.vi"("CAN卡类型"=w6030, "设备索引号"=w6031, "CAN端口"=w6032, "操作类型"=enum16{"初始化CAN", "关闭CAN"}."初始化CAN", "滤波方式"=w6035, "Accept Code"=u32 606601216, "簇"=T23 {"打开CAN"=FALSE, "初始化CAN"=TRUE, "开始CAN"=TRUE, "重启"=FALSE, "关闭CAN"=FALSE}, "Mask Code"=u32 524287 ("Accept Code"), "工作方式"=w6036, "是否滤波"=TRUE, "滤波选择"=T22 {"fiter_mode"=1, "fiter_endid"=75825152, "fiter_startid"=75890687}) -> ()  [unwired: 3 in, 6 out]
              n4228 = Wait Until Next ms Multiple(millisecond multiple=u32 20 ("毫秒倍数")) -> ()  [unwired: 1 out]
            }
            frame #1 {
              n4229 = local read "强制类型"() -> (w6063:enum16{"全通道开启", "单通道开启", "清待均衡时间"})
              n4230 = case shown="\"清待均衡时间\"" w6063 {
                tunnel: [250 252 254] -> w6053
                tunnel: [_ w6082 _] -> w6052
                tunnel: [_ w6081 _] -> w6051
                tunnel: [_ w6072 _] -> w6050
                tunnel: [_ w6065 _] -> w6049
                frame "全通道开启", Default {
                }
                frame "单通道开启" {
                  n4231 = local read "均衡类型选择"() -> (w6080:enum16{"放电均衡", "充电均衡", "充放电均衡"})
                  n4232 = local read "均衡位置"() -> (w6075:u16)
                  n4233 = case shown="\"放电均衡\", 默认" w6080 {
                    tunnel: [0 1] -> w6079
                    frame "放电均衡", Default {
                    }
                    frame "充电均衡" {
                    }
                  }
                  n4234 = Multiply(x="均衡时间", y=6.0) -> (x*y=w6067:dbl)
                  n4235 = Quotient & Remainder(x=w6067, y=256.0) -> (x-y*floor(x/y)=w6065:dbl, floor(x/y)=w6066:dbl)
                  n4236 = call "二进制解析-8.6.vi"("索引"=1, "数值"=w6079) -> ("低位子数组"=w6070:i32[])  [unwired: 1 in, 2 out]
                  n4237 = Quotient & Remainder(x=w6075, y=256.0) -> (x-y*floor(x/y)=w6081:dbl, floor(x/y)=w6082:dbl)
                  n4238 = call "二进制解析-8.6.vi"("索引"=8, "数值"=w6066) -> ("低位子数组"=w6071:i32[])  [unwired: 1 in, 2 out]
                  n4239 = Replace Array Subset(array=w6071, new element=w6070, index=0 ("索引")) -> (w6068:i32[])
                  n4240 = call "数值二进制转十进制-8.6.vi"("子数组"=w6068) -> ("十进制数值"=w6072:i32)  [unwired: 4 in]
                }
                frame "清待均衡时间" {
                }
              }
              n4241 = local write "命令"(w6057) -> ()
              n4242 = call "ID组合.vi"("SA(4)"=0 ("PDU(1)"), "PS(3)"=63 ("PDU(1)"), "PF(2)"=w6057, "PDU(1)"=4) -> ("ID"=w6056:i32)  [unwired: 7 out]
              n4243 = local read "设备索引号"() -> (w6060:u16)
              n4244 = local read "CAN卡类型"() -> (w6061:u32)
              n4245 = local read "CAN端口"() -> (w6059:u16)
              n4246 = local write "命令序号"(w6053) -> ()
              n4247 = Build Array(6, 4, w6053, w6052, w6051, w6050, w6049) -> (w6062:dbl[])
              n4248 = call "transmit-8.6.vi"("can卡类型"=w6061, "设备索引号"=w6060, "CAN端口"=w6059, "ID"=w6056, "SendType"=u8 0, "Data"=w6062) -> ()  [unwired: 3 in, 11 out]
            }
            frame #2 {
              n4249 = Wait Until Next ms Multiple(millisecond multiple=u32 1000 ("毫秒倍数")) -> ()  [unwired: 1 out]
            }
            frame #3 {
              w6096 = u8 0 items=["Normal", "Listen Only"] ("工作方式")
              w6095 = u8 1 items=["Dual Filter", "Single Filter"] ("滤波方式")
              n4250 = global write "EV05全局变量1.vi" "流控帧 2"(FALSE ("流控帧 2")) -> ()
              n4251 = local write "控制1"(FALSE ("控制1")) -> ()
              n4252 = local read "设备索引号"() -> (w6091:u16)
              n4253 = local read "CAN卡类型"() -> (w6090:u32)
              n4254 = local write "消除"(FALSE ("消除")) -> ()
              n4255 = local read "CAN端口"() -> (w6092:u16)
              n4256 = call <vilib>:"Unset Busy.vi"() -> ()  [unwired: 2 in, 10 out]
              n4257 = call "CAN_Init-8.6.vi"("CAN卡类型"=w6090, "设备索引号"=w6091, "CAN端口"=w6092, "操作类型"=enum16{"初始化CAN", "关闭CAN"}."初始化CAN", "滤波方式"=w6095, "Accept Code"=u32 3221225472, "簇"=T23 {"打开CAN"=FALSE, "初始化CAN"=TRUE, "开始CAN"=TRUE, "重启"=FALSE, "关闭CAN"=FALSE}, "Mask Code"=u32 1073741823 ("Accept Code"), "工作方式"=w6096, "是否滤波"=TRUE, "滤波选择"=T22 {"fiter_mode"=1, "fiter_endid"=402653184, "fiter_startid"=419430399}) -> ()  [unwired: 3 in, 6 out]
            }
          }
        }
        frame "项目软件版本读取" {
          n4258 = stacked-sequence {
            seq-local: [_ w6117 _] -> [_ _ w6124]
            frame #0 {
              n4259 = local read "设备索引号"() -> (w6104:u16)
              n4260 = local read "CAN卡类型"() -> (w6105:u32)
              n4261 = local read "CAN端口"() -> (w6103:u16)
              n4262 = stacked-sequence {
                tunnel: w6105 -> [w6108 w6116]
                tunnel: w6104 -> [w6107 w6115]
